vi "Set Multiple Operations.vi"(8 "error in (no error)":errorcluster, 10 "Data":variant[](array[variant]), 11 "Command":string[](array[string])) -> (0 "error out":errorcluster)   [LabVIEW 2014]
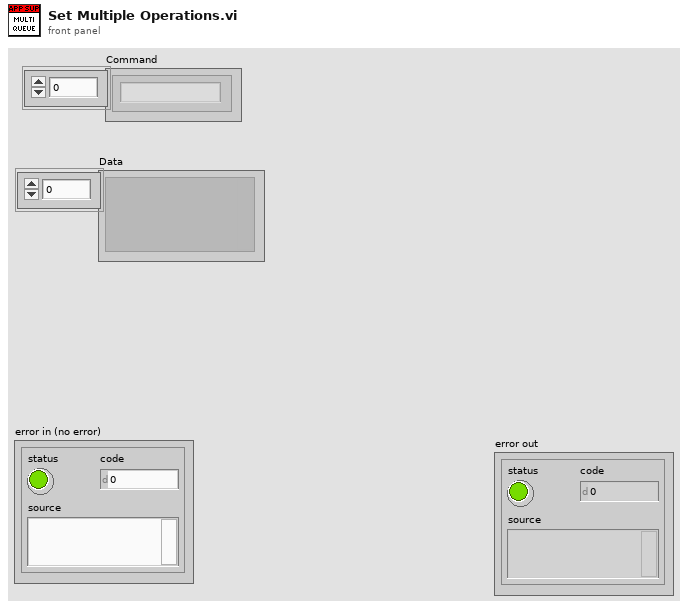
[diagram p1: front panel]
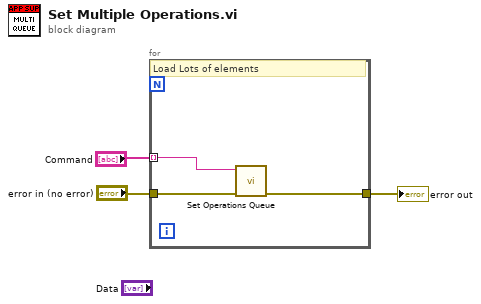
[diagram p0: block diagram]
diagram:
  n1 = for {
    tunnel: "error in (no error)" -> [w6]
    tunnel: [w5] -> w2
    tunnel: "Command" -> [w4] mode=indexing
    # "Load Lots of elements"
    n2 = call "Set Operations Queue.vi"("error in (no error)"=w6, "Command"=w4) -> ("error out"=w5:errorcluster)  [unwired: 9 in]
  }
  "error out" <- w2
